vi "Sway_I2C_2_MPUsV00A.vi"() -> ()   [LabVIEW 2016]
uses:
  <vilib>/MakerHub/LINX/Private/Type Defs/Interface.ctl
  <vilib>/MakerHub/LINX/Public/Sensors/Accelerometer/MPU60X0/Clock Source.ctl
  Control 1.ctl
  <vilib>/MakerHub/LINX/Private/Type Defs/User Platform.ctl
  <vilib>/MakerHub/LINX/Public/Sensors/Accelerometer/MPU60X0/DeviceAddresses.ctl
  <vilib>/MakerHub/LINX/Public/Sensors/Accelerometer/MPU60X0/AccelFullScaleRanges.ctl
  <vilib>/MakerHub/LINX/Public/Sensors/Accelerometer/MPU60X0/GyroFullScaleRanges.ctl
  <vilib>/MakerHub/LINX/Public/Initialize.vi
  <vilib>/MakerHub/LINX/LMH-LINX.lvlib
  <vilib>/MakerHub/LINX/Public/Sensors/Accelerometer/MPU60X0/MPU60X0.lvlib
  <vilib>/Platform/NI_3dgraph.lvlib
panel:
  in  "Baud Rate Override":T1
  in  "Clock Source 2":T2
  out "Waveform kk 2":T3(graph)
  out "Waveform kk":T3(graph)
  out "Path Length":dbl
  out "vector error":errorcluster
  in  "Plot of roll and pitch":refnum<k7>(container)
  out "XY Graph":cluster{"Y":dbl[], "Y":dbl[]}[](graph)
  out "error out":errorcluster
  out "MATLAB Error":errorcluster
  out "Error Out":errorcluster
  in  "?":bool
  in  "I2C Channel":u8
  in  "Clock Source":T2
  in  "Interface":T4
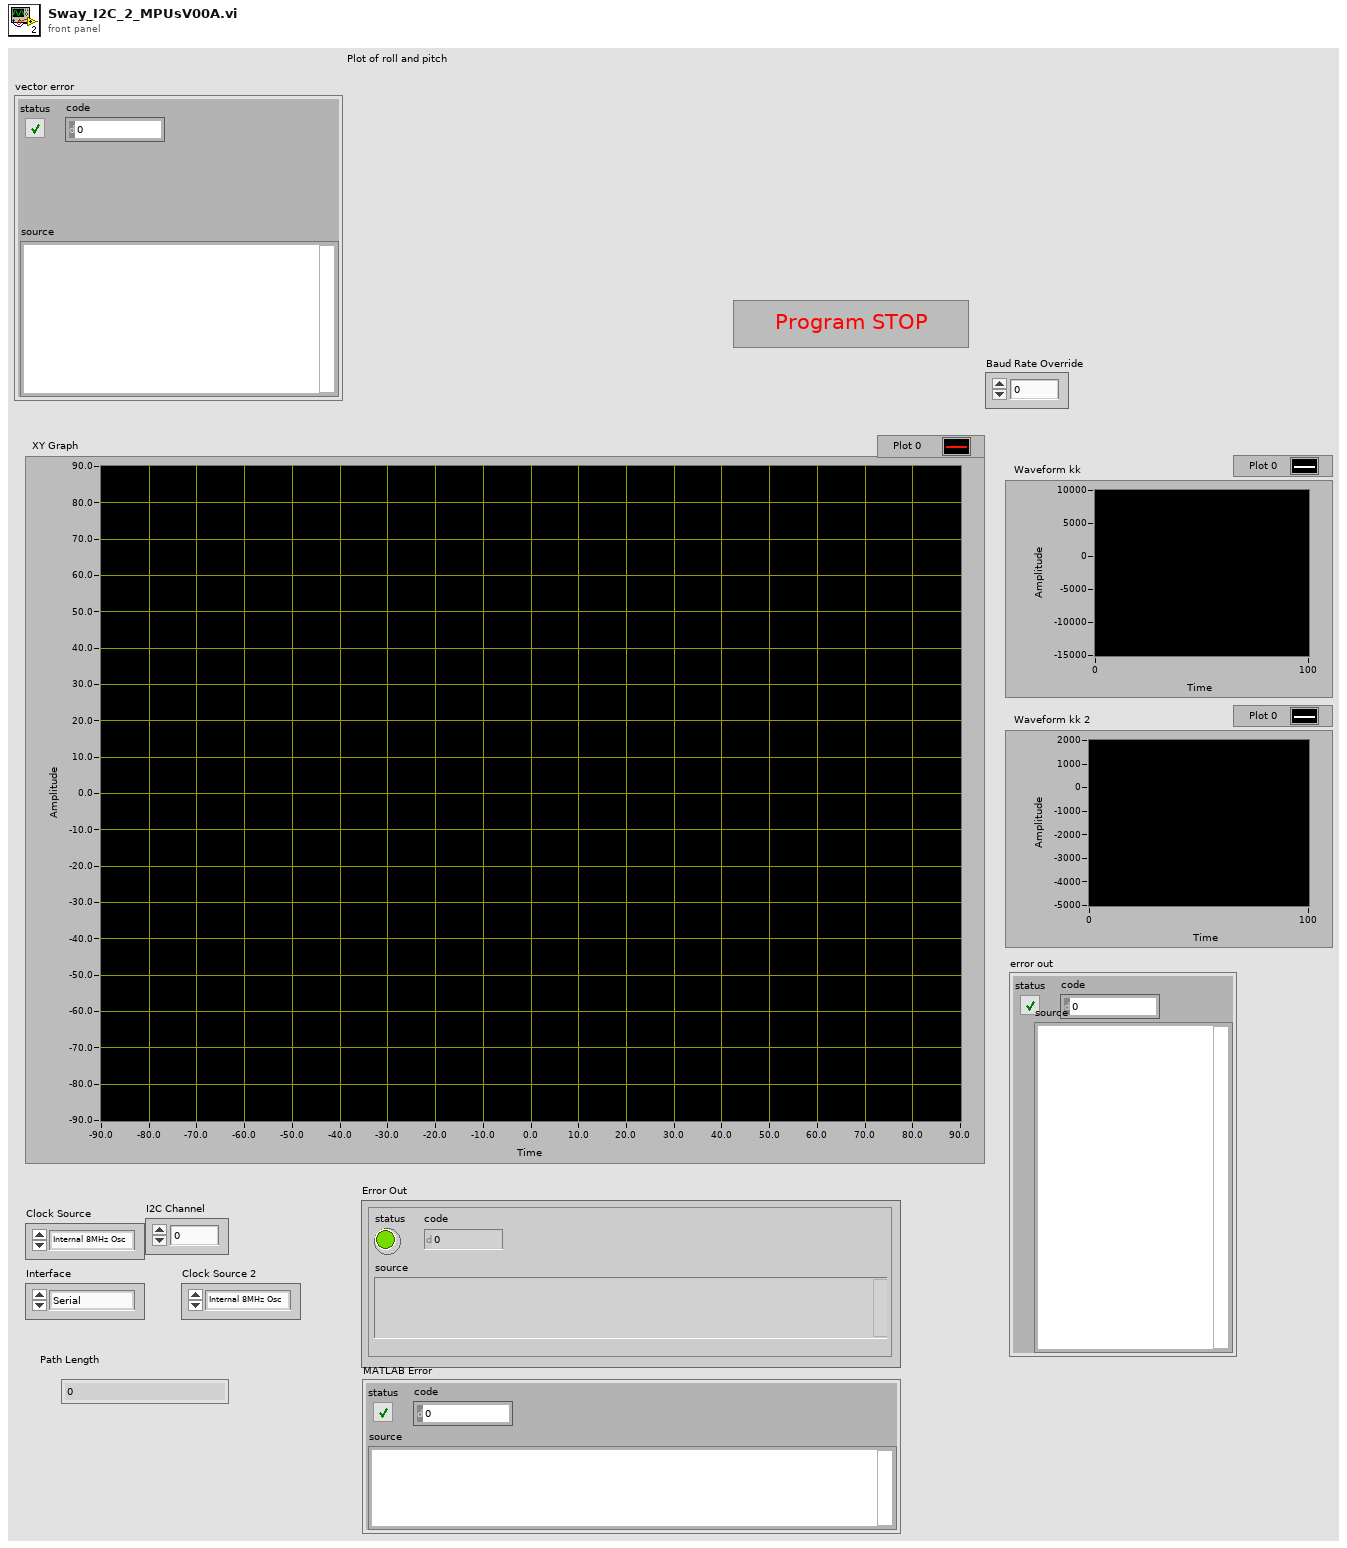
[diagram p1: front panel]
types:
  T1 = typedef "Control 1.ctl" = u32
  T2 = typedef "LMH-LINX.lvlib/MPU60X0.lvlib/Clock Source.ctl" = enum8{"Internal 8MHz Osc", "PLL with X Gyro Ref", "PLL with Y Gyro Ref", "PLL with Z Gyro Ref", "PLL with ext 32.768 KHz Ref", "PLL with ext 19.2 MHz Ref", "Reserved", "Hold in reset"}
  T3 = cluster{"X Axis":i16, "Y Axis":i16, "Z Axis":i16}
  T4 = typedef "LMH-LINX.lvlib/Interface.ctl" = enum16{"Serial", "TCP"}
  T5 = typedef "LMH-LINX.lvlib/MPU60X0.lvlib/DeviceAddresses.ctl" = enum16{"0x68", "0x69"}
  T6 = typedef "LMH-LINX.lvlib/MPU60X0.lvlib/GyroFullScaleRanges.ctl" = enum8{"±250 °/s", "±500 °/s", "±1000 °/s", "±2000 °/s"}
  T7 = typedef "LMH-LINX.lvlib/MPU60X0.lvlib/AccelFullScaleRanges.ctl" = enum16{"±2g", "±4g", "±8g", "±16g"}
  T8 = typedef "LMH-LINX.lvlib/User Platform.ctl" = enum16{"Default", "Remote", "Local"}
  T9 = typedef "LMH-LINX.lvlib/LINX Ref.ctl" = cluster{"IO":T10, "Interface":T4, "LINX Device Config":T11}
  T10 = typedef "LMH-LINX.lvlib/Platform.ctl" = enum16{"Remote", "Local"}
  T11 = typedef "LMH-LINX.lvlib/Device.lvlib/LINX Device Config.ctl" = cluster{"Interface":T4, "COM Port":refnum<visa-resource-name>, "TCP Configuration":T12, "Device Family":u8, "Device ID":u8, "Device Name":string, "TCP Ref":refnum<k5>, "Channels":T13}
  T12 = typedef "LMH-LINX.lvlib/Device.lvlib/TCP Config.ctl" = cluster{"IP Address":string, "Port":u16}
  T13 = typedef "LMH-LINX.lvlib/Channels.ctl" = cluster{"DI":u8[], "DO":u8[], "AI":u8[], "AO":u8[], "PWM":u8[], "QE":u8[], "UART":u8[], "I2C 2":u8[], "SPI":u8[], "CAN":u8[], "Servo":u8[], "AI Ref (V)":dbl, "AI Resolution (Bits)":u8, "AO Ref (V)":dbl, "AO Resolution (Bits)":u8}
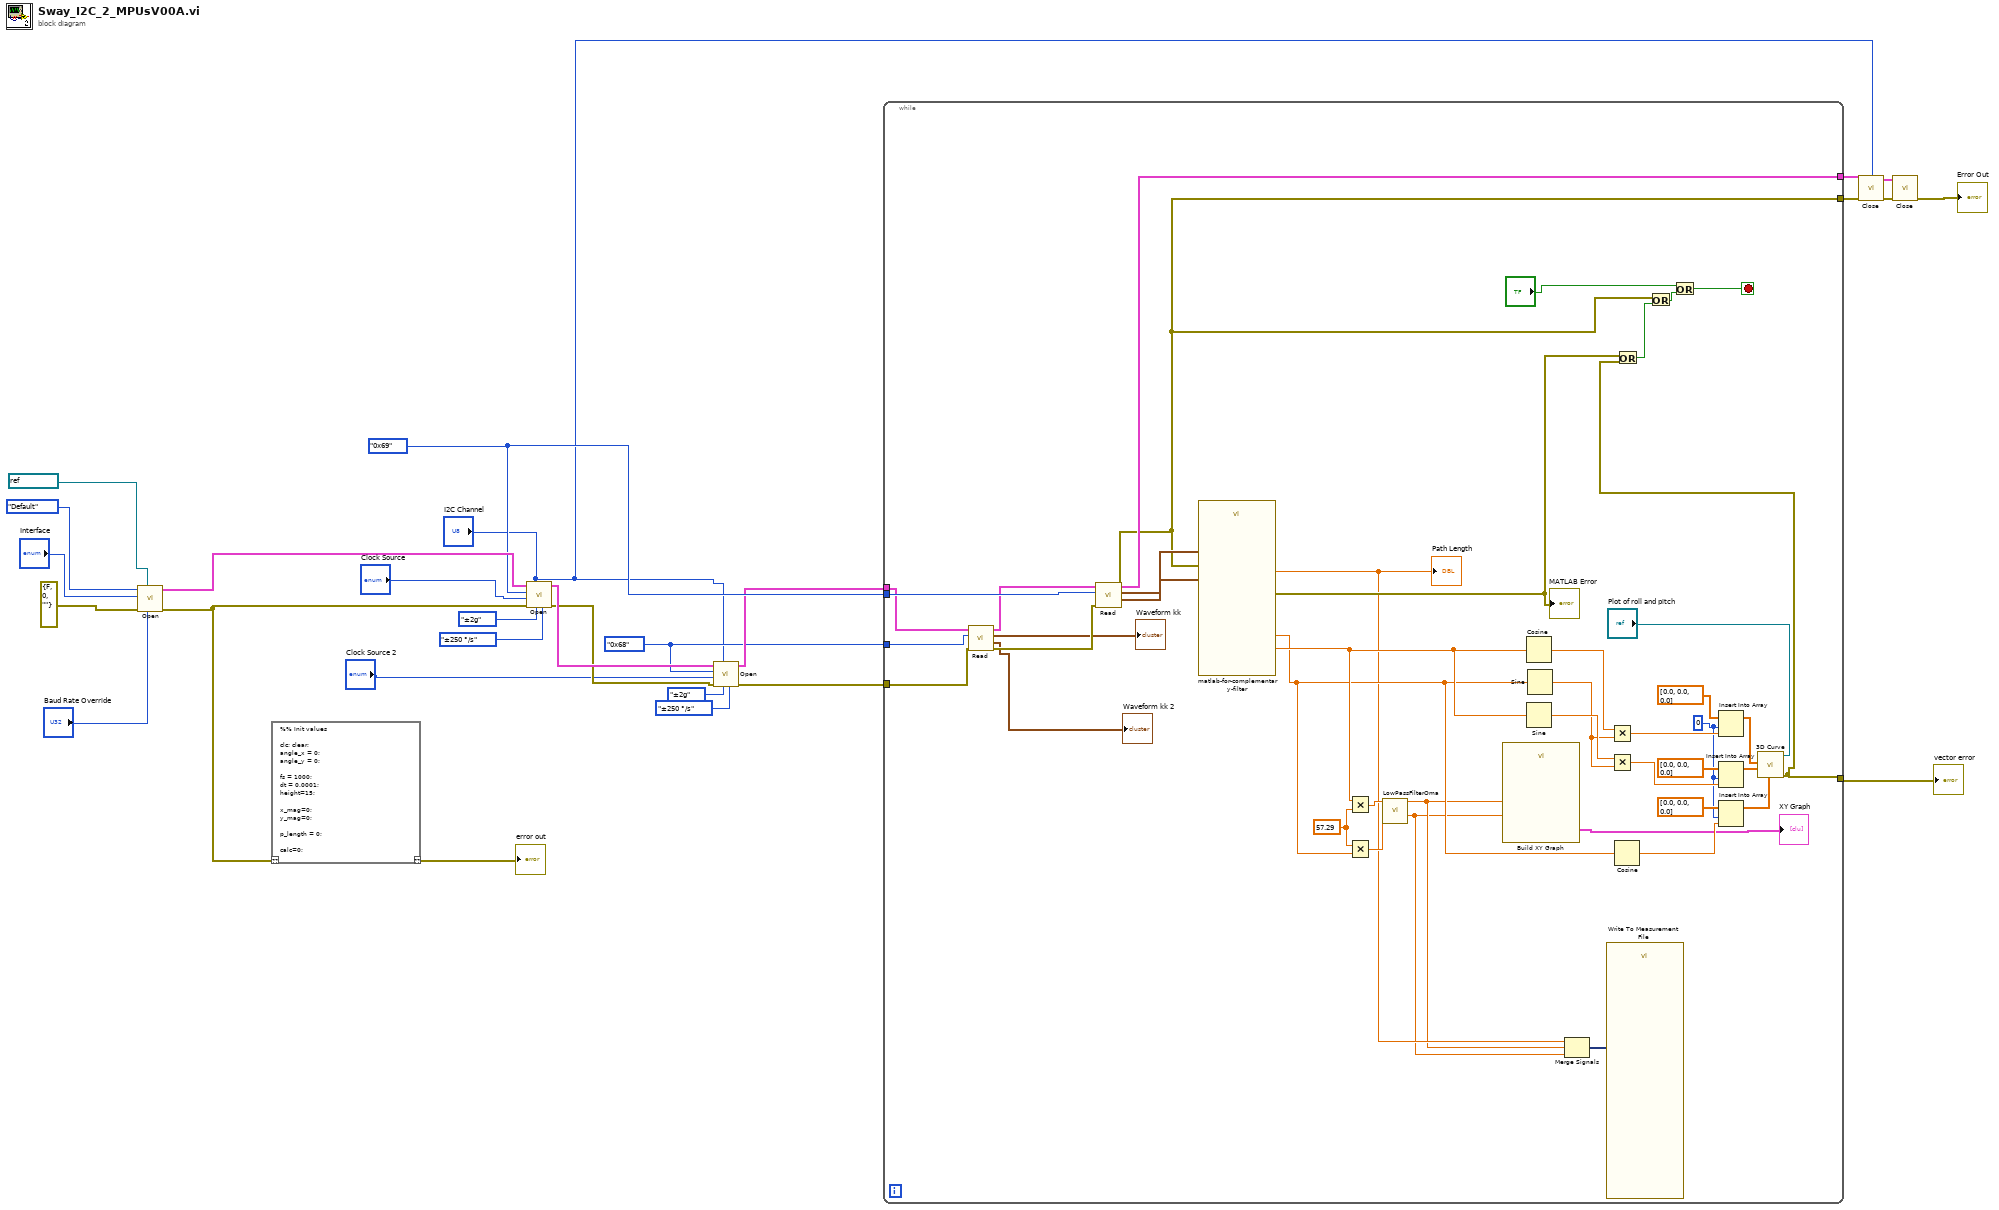
[diagram p0: block diagram]
diagram:
  w5 = DeviceAddresses."0x68" ("I2C Slave Address")
  w22 = DeviceAddresses."0x69" ("Device Address")
  n1 = call-poly <vilib>:"Open.vi"("Baud Rate Override"="Baud Rate Override", "Serial Port"=refnum<visa-resource-name> "COM3", "Error In"=errorcluster {"status"=FALSE, "code"=0, "source"=""}, "Interface"="Interface", "IO"=User_Platform."Default") -> ("Error Out"=w16:errorcluster, "LINX Resource"=w25:T9)  [unwired: 4 in, 1 out]
  n2 = script code="%% Init values\n\nclc; clear;\nangle_x = 0;\nangle_y = 0;\n\nfs = 1000;\ndt = 0.0001;\nheight=15;\n\nx_mag=0; \ny_mag=0; \n\np_length = 0;\n\ncalc=0;"("??"=w16) -> ("??"=→"error out":errorcluster)
  n3 = call <vilib>:"Open.vi"("Gyro Full Scale Range"=GyroFullScaleRanges."±250 °/s", "Accel Full Scale Range"=AccelFullScaleRanges."±2g", "I2C Channel"="I2C Channel", "Error In"=w16, "Clock Source"="Clock Source", "I2C Slave Address"=w22, "LINX Resource"=w25) -> ("Error Out"=w7:errorcluster, "LINX Resource"=w11:T9)  [unwired: 3 in]
  n4 = call <vilib>:"Open.vi"("Gyro Full Scale Range"=GyroFullScaleRanges."±250 °/s", "Accel Full Scale Range"=AccelFullScaleRanges."±2g", "I2C Channel"="I2C Channel", "Error In"=w7, "Clock Source"="Clock Source 2", "I2C Slave Address"=w5, "LINX Resource"=w11) -> ("Error Out"=w6:errorcluster, "LINX Resource"=w10:T9)  [unwired: 3 in]
  n5 = while {
    tunnel: w10 -> [w40]
    tunnel: w22 -> [w69]
    tunnel: [w68] -> w21
    tunnel: [w44] -> w19
    tunnel: [w45] -> w12
    tunnel: w6 -> [w37]
    tunnel: w5 -> [w38]
    stop <- w48 stop-if-true
    w52 = 57.29 ("y")
    w54 = 0 ("index")
    n6 = call <vilib>:"Read.vi"("Error In"=w37, "I2C Slave Address"=w38, "LINX Resource"=w40) -> ("Error Out"=w36:errorcluster, "Gyro  Data (dps)"=→"Waveform kk 2":T3, "Acceleration Data (g)"=→"Waveform kk":T3, "LINX Resource"=w39:T9)  [unwired: 4 in, 1 out]
    n7 = call <vilib>:"Read.vi"("Error In"=w36, "I2C Slave Address"=w69, "LINX Resource"=w39) -> ("Error Out"=w44:errorcluster, "Gyro  Data (dps)"=w66:T3, "Acceleration Data (g)"=w67:T3, "LINX Resource"=w68:T9)  [unwired: 4 in, 1 out]
    n8 = call "matlab-for-complementary-filter.vi"("Acceleration Data (g)"=w67, "Gyro  Data (dps)"=w66, "error in (no error)"=w44) -> ("angle_y"=w53:dbl, "Path Length"=w30:dbl, "angle_x"=w51:dbl, "error out"=w46:errorcluster)  [unwired: 11 in, 2 out]
    "MATLAB Error" <- w46
    "Path Length" <- w30
    n9 = Multiply(x=w53, y=w52) -> (x*y=w33:dbl)
    n10 = Multiply(x=w52, y=w51) -> (x*y=w32:dbl)
    n11 = call "LowPassFilterOma.vi"("Numeric"=w32, "Numeric 2"=w33) -> ("Filtered x"=w28:dbl, "Filtered x 2"=w29:dbl)  [unwired: 8 in]
    n12 = call "Build XY Graph"("Y Input"=w28, "X Input"=w29) -> ("XY Graph"=→"XY Graph":cluster{"X":dbl[], "Y":dbl[]}[])  [unwired: 8 in, 1 out]
    n13 = Cosine(x=w53) -> (cos(x)=w65:dbl)
    n14 = Sine(x=w53) -> (sin(x)=w60:dbl)
    n15 = Sine(x=w51) -> (sin(x)=w59:dbl)
    n16 = Merge Signals(w30, w29, w28) -> (w31:dynamicdata)
    n17 = call "Write To Measurement File"("Signals"=w31) -> ()  [unwired: 16 in, 3 out]
    n18 = Multiply(x=w65, y=w59) -> (x*y=w62:dbl)
    n19 = Multiply(x=w60, y=w59) -> (x*y=w58:dbl)
    n20 = Cosine(x=w51) -> (cos(x)=w56:dbl)
    n21 = Insert Into Array(array=dbl[] [0.0, 0.0, 0.0], index=w54, new element=w62) -> (w50:dbl[])
    n22 = Insert Into Array(array=dbl[] [0.0, 0.0, 0.0], index=w54, new element=w58) -> (w49:dbl[])
    n23 = Insert Into Array(array=dbl[] [0.0, 0.0, 0.0], index=w54, new element=w56) -> (w55:dbl[])
    n24 = call <vilib>:"3D Curve.vi"("z vector"=w55, "y vector"=w49, "x vector"=w50, "3D graph"="Plot of roll and pitch") -> ("error out"=w45:errorcluster)  [unwired: 6 in, 1 out]
    n25 = Or(x=w46, y=w45) -> (x .or. y?=w47:bool)
    n26 = Or(x=w44, y=w47) -> (x .or. y?=w42:bool)
    n27 = Or(x="?", y=w42) -> (x .or. y?=w48:bool)
  }
  "vector error" <- w12
  n28 = call <vilib>:"Close.vi"("I2C Channel (0)"="I2C Channel", "Error In"=w19, "LINX Resource"=w21) -> ("Error Out"=w18:errorcluster, "LINX Resource"=w20:T9)  [unwired: 7 in]
  n29 = call <vilib>:"Close.vi"("Error In"=w18, "LINX Resource"=w20) -> ("Error Out"=→"Error Out":errorcluster)  [unwired: 9 in]
